vi "Destroy Request Events.vi"(8 "error in":errorcluster) -> (0 "error out":errorcluster)   [LabVIEW 2025, in "Power Supply.lvlib"]
doc: "Destroy the requests user events, even if there is an incoming error.\n\n<b>NOTE</b>: The contents of this VI are automatically generated and modified by the <b>Tools > DQMH Consortium > DQMH</b> utilities. Consider using those utilities instead of making your own modifications to this VI.\n_____\nBased on DQMH Dev Tools: Project Template 7.1.2.1547."
uses:
  Power Supply.lvlib
panel:
  # "NOTE: The contents of this VI are automatically generated and modified by the Tools > DQMH Consortium > DQMH utilities. Consider using those utilities instead of making your own modifications to this VI."
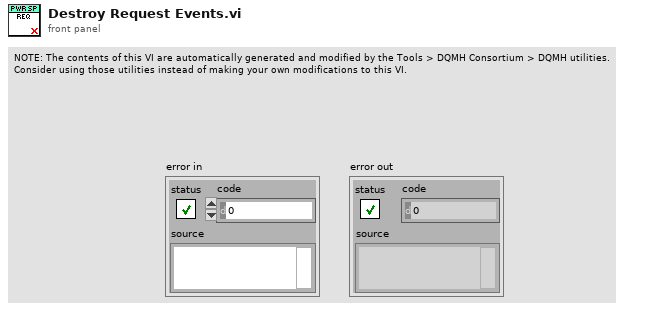
[diagram p1: front panel]
types:
  T1 = typedef "Power Supply.lvlib/Request Events--cluster.ctl" = cluster{"Stop Module":refnum<user-event>, "Show Panel":refnum<user-event>, "Hide Panel":refnum<user-event>, "Show Diagram":refnum<user-event>, "Get Module Execution Status":refnum<user-event>, "select child":refnum<user-event>, "read config":refnum<user-event>, "init device":refnum<user-event>, "close":refnum<user-event>, "output":refnum<user-event>, "set voltage":refnum<user-event>, "set current":refnum<user-event>, "read current":refnum<user-event>, "read voltage":refnum<user-event>, "read state":refnum<user-event>, "set all outputs":refnum<user-event>}
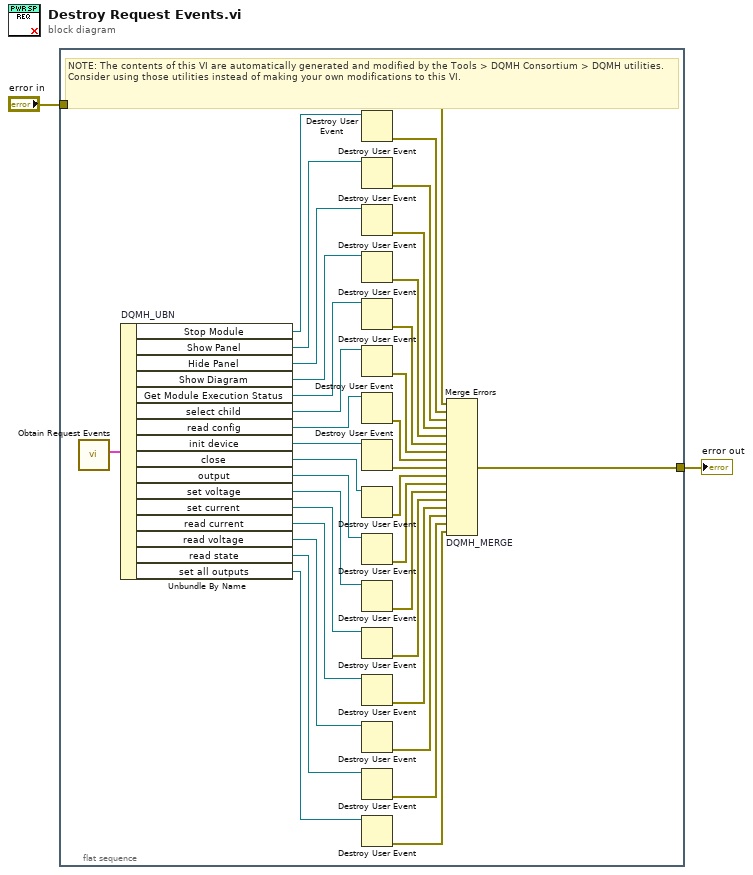
[diagram p0: block diagram]
diagram:
  n1 = flat-sequence {
    tunnel: [w36] -> w2
    tunnel: "error in" -> [w29]
    frame #0 {
      # "NOTE: The contents of this VI are automatically generated and modified by the Tools > DQMH Consortium > DQMH utilities. Consider using those utilities instead of making your own modifications to this VI."
      n2 = call "Obtain Request Events.vi"() -> ("Power Supply Request Events"=w35:T1)  [unwired: 10 in, 1 out]
      n3 = Unbundle By Name "DQMH_UBN"(w35) -> ("Stop Module"=w34:refnum<user-event>, "Show Panel"=w31:refnum<user-event>, "Hide Panel"=w30:refnum<user-event>, "Show Diagram"=w27:refnum<user-event>, "Get Module Execution Status"=w25:refnum<user-event>, "select child"=w23:refnum<user-event>, "read config"=w21:refnum<user-event>, "init device"=w19:refnum<user-event>, "close"=w17:refnum<user-event>, "output"=w15:refnum<user-event>, "set voltage"=w13:refnum<user-event>, "set current"=w11:refnum<user-event>, "read current"=w9:refnum<user-event>, "read voltage"=w7:refnum<user-event>, "read state"=w5:refnum<user-event>, "set all outputs"=w3:refnum<user-event>)
      n4 = Destroy User Event(user event=w34) -> (error out=w37:errorcluster)  [unwired: 1 in]
      n5 = Destroy User Event(user event=w31) -> (error out=w33:errorcluster)  [unwired: 1 in]
      n6 = Destroy User Event(user event=w30) -> (error out=w32:errorcluster)  [unwired: 1 in]
      n7 = Destroy User Event(user event=w27) -> (error out=w28:errorcluster)  [unwired: 1 in]
      n8 = Destroy User Event(user event=w25) -> (error out=w26:errorcluster)  [unwired: 1 in]
      n9 = Destroy User Event(user event=w23) -> (error out=w24:errorcluster)  [unwired: 1 in]
      n10 = Destroy User Event(user event=w21) -> (error out=w22:errorcluster)  [unwired: 1 in]
      n11 = Destroy User Event(user event=w19) -> (error out=w20:errorcluster)  [unwired: 1 in]
      n12 = Destroy User Event(user event=w17) -> (error out=w18:errorcluster)  [unwired: 1 in]
      n13 = Destroy User Event(user event=w15) -> (error out=w16:errorcluster)  [unwired: 1 in]
      n14 = Destroy User Event(user event=w13) -> (error out=w14:errorcluster)  [unwired: 1 in]
      n15 = Destroy User Event(user event=w11) -> (error out=w12:errorcluster)  [unwired: 1 in]
      n16 = Destroy User Event(user event=w9) -> (error out=w10:errorcluster)  [unwired: 1 in]
      n17 = Destroy User Event(user event=w7) -> (error out=w8:errorcluster)  [unwired: 1 in]
      n18 = Destroy User Event(user event=w5) -> (error out=w6:errorcluster)  [unwired: 1 in]
      n19 = Destroy User Event(user event=w3) -> (error out=w4:errorcluster)  [unwired: 1 in]
      n20 = Merge Errors "DQMH_MERGE"(w29, w37, w33, w32, w28, w26, w24, w22, w20, w18, w16, w14, w12, w10, w8, w6, w4) -> (w36:errorcluster)
    }
  }
  "error out" <- w2
